vi "PH_ToImage.vi"(0 "Data In":u32[](array[numeric]), 1 "Reset":bool, 2 "Image Array In":i32[][](array[numeric]), 5 "Data Count":i32, 9 "Pixel Time (Laser Pulses)":i32=25, 11 "Trace Bins":i32=25) -> (3 "Image Array Out":i32[][](array[numeric]), 4 "Histograms":i32[][](array[numeric]), 6 "Total Photon Count":u64[](array[numeric]), 8 "Trigger Times":u64[](array[numeric]), 13 "Total Oveflow Count":u64, 14 "Num Records Total":i32, 15 "Traces":i32[][](array[numeric]))   [LabVIEW 2010]
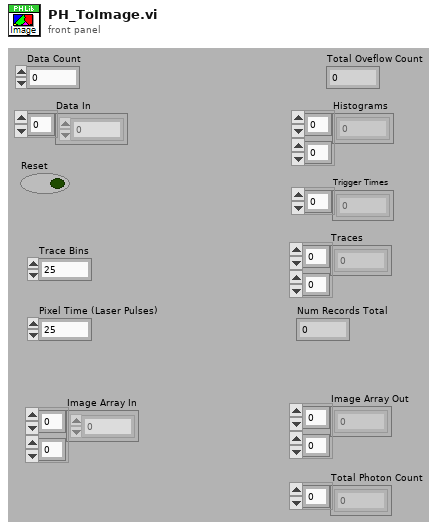
[diagram p1: front panel]
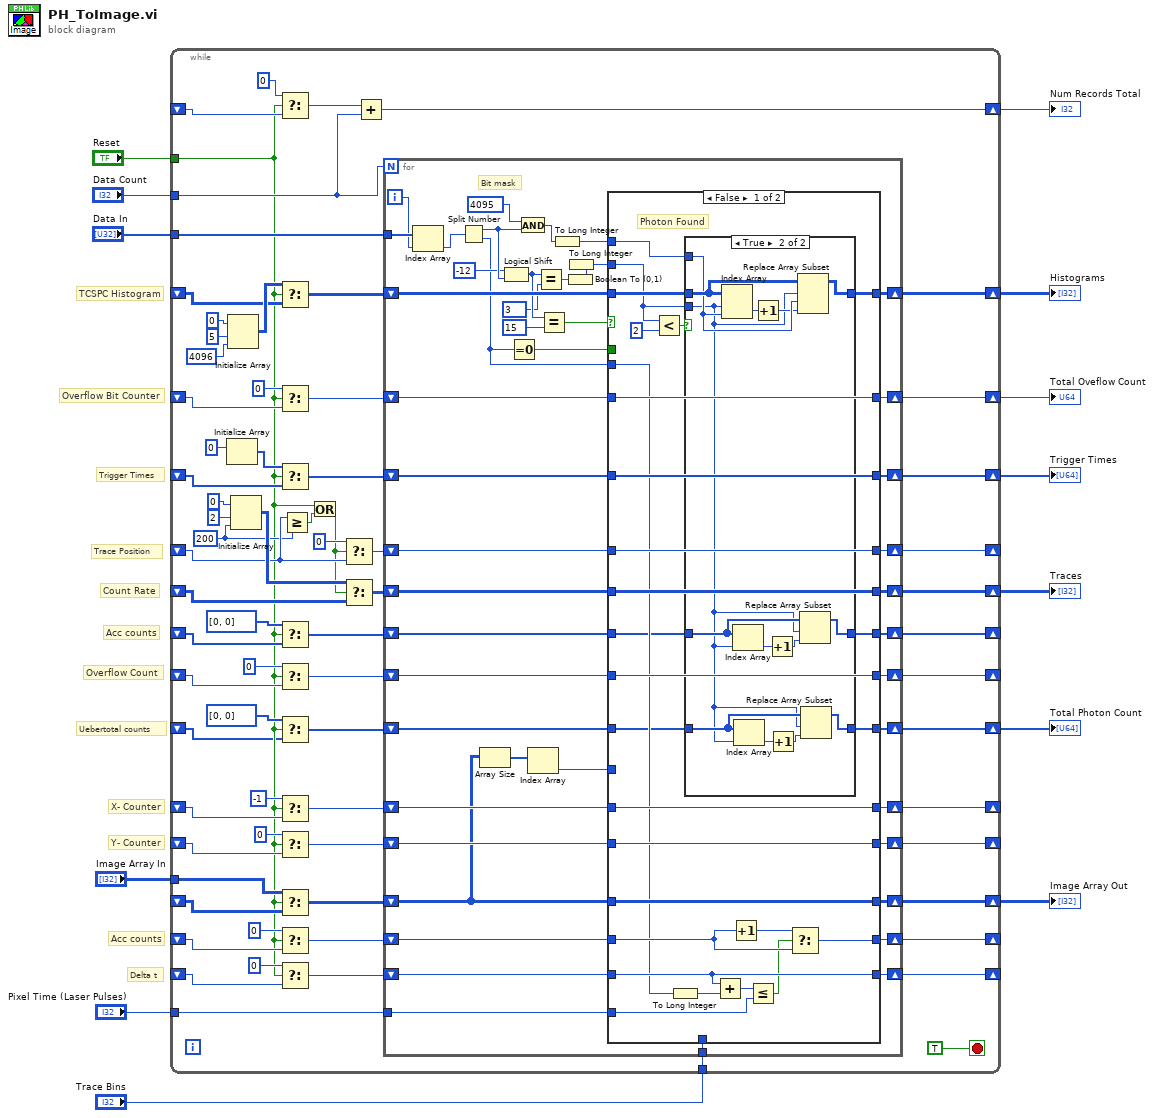
[diagram p0: block diagram]
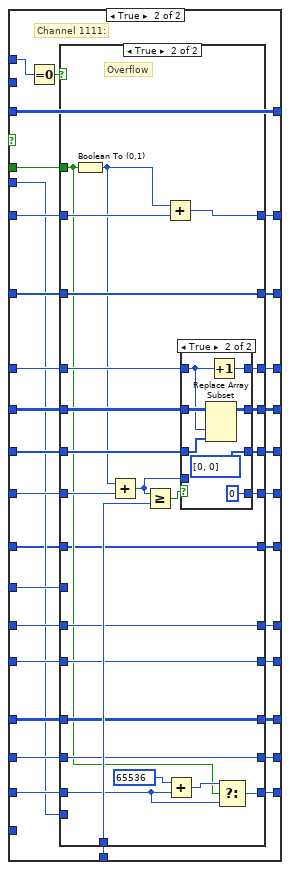
[diagram p3: hidden frame]
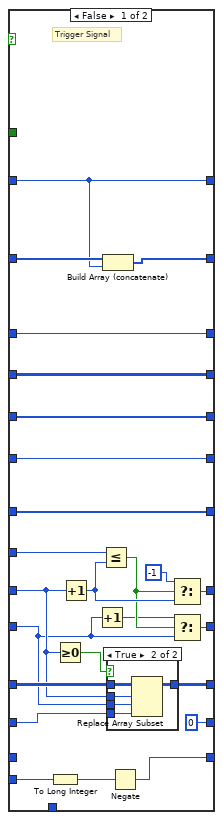
[diagram p4: hidden frame]
diagram:
  # "Uebertotal counts"
  # "Y- Counter"
  # "X- Counter"
  # "Delta t"
  # "Acc counts"
  # "Trace Position"
  # "Overflow Count"
  # "Acc counts"
  # "Count Rate"
  # "Trigger Times"
  # "TCSPC Histogram"
  # "Overflow Bit Counter"
  n1 = while {
    tunnel: "Data In" -> [w82]
    shift-right: [w83] -> w13
    shift-left: _ -> [w78]
    tunnel: "Reset" -> [w17]
    shift-right: [w75] -> w2
    shift-left: _ -> [w74]
    shift-right: [w70] -> w10
    shift-left: _ -> [w69]
    shift-right: [w65] -> w8
    shift-left: _ -> [w64]
    shift-right: [w62] -> _
    shift-left: _ -> [w61]
    shift-right: [w59] -> _
    shift-left: _ -> [w58]
    tunnel: "Trace Bins" -> [w57]
    shift-right: [w54] -> _
    shift-left: _ -> [w52]
    shift-right: [w48] -> w5
    shift-left: _ -> [w47]
    tunnel: "Image Array In" -> [w50]
    shift-right: [w43] -> _
    shift-left: _ -> [w41]
    shift-right: [w42] -> _
    shift-left: _ -> [w40]
    tunnel: "Pixel Time (Laser Pulses)" -> [w39]
    shift-right: [w34] -> _
    shift-left: _ -> [w32]
    shift-right: [w33] -> _
    shift-left: _ -> [w31]
    tunnel: "Data Count" -> [w26]
    shift-right: [w25] -> w3
    shift-left: _ -> [w28]
    shift-right: [w15] -> w1
    shift-left: _ -> [w14]
    stop <- TRUE stop-if-true
    w22 = 200 ("dimension size")
    n2 = Initialize Array(u64 0 ("element")) -> (w72:u64[])  [unwired: 1 in]
    n3 = Initialize Array(0 ("element"), 5 ("dimension size"), 4096 ("dimension size")) -> (w79:i32[][])
    n4 = Initialize Array(0 ("element"), 2 ("dimension size"), w22) -> (w67:i32[][])
    n5 = Select(t=0 ("Data Count 2"), s=w17, f=w28) -> (s? t:f=w27:i32)
    n6 = Select(t=w79, s=w17, f=w78) -> (s? t:f=w80:i32[][])
    n7 = Select(t=u64 0, s=w17, f=w74) -> (s? t:f=w76:u64)
    n8 = Select(t=w72, s=w17, f=w69) -> (s? t:f=w71:u64[])
    n9 = Select(t=u32[] [0, 0] ("initialized array"), s=w17, f=w61) -> (s? t:f=w63:u32[])
    n10 = Select(t=u32 0, s=w17, f=w58) -> (s? t:f=w60:u32)
    n11 = Select(t=u64[] [0, 0] ("initialized array"), s=w17, f=w14) -> (s? t:f=w16:u64[])
    n12 = Select(t=-1, s=w17, f=w32) -> (s? t:f=w36:i32)
    n13 = Select(t=0, s=w17, f=w31) -> (s? t:f=w35:i32)
    n14 = Select(t=w50, s=w17, f=w47) -> (s? t:f=w49:i32[][])
    n15 = Select(t=0, s=w17, f=w41) -> (s? t:f=w45:i32)
    n16 = Select(t=0, s=w17, f=w40) -> (s? t:f=w44:i32)
    n17 = Greater Or Equal?(x=w52, y=w22) -> (x >= y?=w53:bool)
    n18 = Or(x=w17, y=w53) -> (x .or. y?=w51:bool)
    n19 = Select(t=0, s=w51, f=w52) -> (s? t:f=w55:i32)
    n20 = Select(t=w67, s=w51, f=w64) -> (s? t:f=w66:i32[][])
    n21 = Add(x=w27, y=w26) -> (x+y=w25:i32)
    n22 = for {
      N: w26 -> [_]
      tunnel: w82 -> [w94]
      shift-right: [w127] -> w83
      shift-left: w80 -> [w129]
      shift-right: [w121] -> w75
      shift-left: w76 -> [w122]
      shift-right: [w119] -> w70
      shift-left: w71 -> [w120]
      shift-right: [w114] -> w65
      shift-left: w66 -> [w115]
      shift-right: [w116] -> w62
      shift-left: w63 -> [w117]
      shift-right: [w112] -> w59
      shift-left: w60 -> [w113]
      tunnel: w57 -> [w111]
      shift-right: [w109] -> w54
      shift-left: w55 -> [w110]
      shift-right: [w108] -> w48
      shift-left: w49 -> [w100]
      shift-right: [w106] -> w43
      shift-left: w45 -> [w107]
      shift-right: [w104] -> w42
      shift-left: w44 -> [w105]
      tunnel: w39 -> [w96]
      shift-right: [w101] -> w34
      shift-left: w36 -> [w102]
      shift-right: [w97] -> w33
      shift-left: w35 -> [w103]
      shift-right: [w85] -> w15
      shift-left: w16 -> [w86]
      i -> [w93]
      # "Bit mask"
      n23 = Index Array(array=w94, index=w93) -> (element=w92:u32)
      n24 = Split Number(x=w92) -> (hi(x)=w126:u16, lo(x)=w95:u16)
      n25 = Array Size(array=w100) -> (size(s)=w99:i32[])
      n26 = Logical Shift(y=i8 -12, x=w126) -> (x << y=w91:u16)
      n27 = Equal To 0?(x=w95) -> (x = 0?=w118:bool)
      n28 = And(x=u16 4095, y=w126) -> (x .and. y?=w130:u16)
      n29 = Index Array(array=w99) -> (element=w98:i32)  [unwired: 1 in]
      n30 = Equal?(x=w91, y=u16 3) -> (x = y?=w89:bool)
      n31 = Equal?(x=w91, y=u16 15) -> (x = y?=w123:bool)
      n32 = To Long Integer(number=w130) -> (32bit integer=w128:i32)
      n33 = Boolean To (0,1)(Boolean=w89) -> (0, 1=w88:i16)
      n34 = To Long Integer(number=w88) -> (32bit integer=w87:i32)
      n35 = case shown="False" w123 {
        tunnel: w129 -> [w158 w203]
        tunnel: w128 -> [w139 w184]
        tunnel: [w157 w203] -> w127
        tunnel: w87 -> [w135 _]
        tunnel: w122 -> [w156 w205]
        tunnel: [w156 w204] -> w121
        tunnel: w120 -> [w155 w202]
        tunnel: [w155 w201] -> w119
        tunnel: w118 -> [_ w200]
        tunnel: w117 -> [w138 w198]
        tunnel: [w137 w194] -> w116
        tunnel: w115 -> [w154 w197]
        tunnel: [w154 w193] -> w114
        tunnel: w113 -> [w153 w199]
        tunnel: [w153 w195] -> w112
        tunnel: w111 -> [_ w196]
        tunnel: w110 -> [w152 w192]
        tunnel: [w152 w191] -> w109
        tunnel: w100 -> [w151 w189]
        tunnel: [w151 w190] -> w108
        tunnel: w107 -> [w150 w185]
        tunnel: [w149 w186] -> w106
        tunnel: w105 -> [w148 w188]
        tunnel: [w148 w187] -> w104
        tunnel: w103 -> [w147 w183]
        tunnel: w102 -> [w146 w182]
        tunnel: [w146 w181] -> w101
        tunnel: w98 -> [_ w180]
        tunnel: [w147 w179] -> w97
        tunnel: w96 -> [w145 _]
        tunnel: w95 -> [w141 w178]
        tunnel: w86 -> [w133 w177]
        tunnel: [w132 w176] -> w85
        frame False {
          # "Photon Found"
          n36 = Less?(x=w135, y=2) -> (x < y?=w136:bool)
          n37 = To Long Integer(number=w141) -> (32bit integer=w140:i32)
          n38 = case shown="True" w136 {
            tunnel: w158 -> [w161 w175]
            tunnel: [w161 w174] -> w157
            tunnel: w139 -> [_ w173]
            tunnel: w135 -> [_ w162]
            tunnel: w138 -> [w160 w172]
            tunnel: [w160 w171] -> w137
            tunnel: w133 -> [w159 w164]
            tunnel: [w159 w163] -> w132
            frame False {
            }
            frame True {
              n39 = Index Array(array=w175, index (row)=w162, index (col)=w173) -> (element=w170:i32)
              n40 = Index Array(array=w172, index=w162) -> (element=w168:u32)
              n41 = Index Array(array=w164, index=w162) -> (element=w166:u64)
              n42 = Increment(x=w170) -> (x+1=w169:i32)
              n43 = Increment(x=w168) -> (x+1=w167:u32)
              n44 = Increment(x=w166) -> (x+1=w165:u64)
              n45 = Replace Array Subset(array=w175, new element=w169, index (row)=w162, index (col)=w173) -> (w174:i32[][])
              n46 = Replace Array Subset(array=w172, new element=w167, index=w162) -> (w171:u32[])
              n47 = Replace Array Subset(array=w164, new element=w165, index=w162) -> (w163:u64[])
            }
          }
          n48 = Add(x=w148, y=w140) -> (x+y=w142:i32)
          n49 = Increment(x=w150) -> (x+1=w144:i32)
          n50 = Less Or Equal?(x=w142, y=w145) -> (x <= y?=w143:bool)
          n51 = Select(t=w144, s=w143, f=w150) -> (s? t:f=w149:i32)
        }
        frame True {
          # "Channel 1111:"
          n52 = Equal To 0?(x=w184) -> (x = 0?=w206:bool)
          n53 = case shown="True" w206 {
            tunnel: w205 -> [w229 w261]
            tunnel: [w229 w260] -> w204
            tunnel: w202 -> [w231 w262]
            tunnel: [w230 w262] -> w201
            tunnel: w200 -> [_ w239]
            tunnel: w199 -> [w228 w245]
            tunnel: w198 -> [w227 w256]
            tunnel: w197 -> [w226 w254]
            tunnel: w196 -> [_ w259]
            tunnel: [w228 w257] -> w195
            tunnel: [w227 w255] -> w194
            tunnel: [w226 w253] -> w193
            tunnel: w192 -> [w225 w252]
            tunnel: [w225 w251] -> w191
            tunnel: [w222 w250] -> w190
            tunnel: w189 -> [w223 w250]
            tunnel: w188 -> [_ w240]
            tunnel: [w208 w241] -> w187
            tunnel: [0 ("t") w248] -> w186
            tunnel: w185 -> [w221 w248]
            tunnel: w178 -> [w224 _]
            tunnel: w183 -> [w211 w247]
            tunnel: w182 -> [w216 w246]
            tunnel: [w218 w246] -> w181
            tunnel: w180 -> [w217 _]
            tunnel: [w212 w247] -> w179
            tunnel: w177 -> [w207 w238]
            tunnel: [w207 w238] -> w176
            frame False {
              # "Trigger Signal"
              n54 = To Long Integer(number=w224) -> (32bit integer=w209:i32)
              n55 = Greater Or Equal To 0?(x=w216) -> (x >= 0?=w219:bool)
              n56 = Increment(x=w216) -> (x+1=w215:i32)
              n57 = Increment(x=w211) -> (x+1=w210:i32)
              n58 = Less Or Equal?(x=w217, y=w215) -> (x <= y?=w213:bool)
              n59 = Build Array (concatenate)(w231, w229) -> (w230:u64[])
              n60 = case shown="True" w219 {
                tunnel: w223 -> [w232 w237]
                tunnel: [w232 w236] -> w222
                tunnel: w221 -> [_ w235]
                tunnel: w211 -> [_ w234]
                tunnel: w216 -> [_ w233]
                frame False {
                }
                frame True {
                  n61 = Replace Array Subset(array=w237, new element=w235, index (row)=w233, index (col)=w234) -> (w236:i32[][])
                }
              }
              n62 = Negate(x=w209) -> (-x=w208:i32)
              n63 = Select(t=-1, s=w213, f=w215) -> (s? t:f=w218:i32)
              n64 = Select(t=w210, s=w213, f=w211) -> (s? t:f=w212:i32)
            }
            frame True {
              # "Overflow"
              n65 = Boolean To (0,1)(Boolean=w239) -> (0, 1=w243:i16)
              n66 = Add(x=w243, y=w245) -> (x+y=w244:u32)
              n67 = Greater Or Equal?(x=w244, y=w259) -> (x >= y?=w258:bool)
              n68 = Add(x=w243, y=w261) -> (x+y=w260:u64)
              n69 = Add(x=65536 ("t"), y=w240) -> (x+y=w242:i32)
              n70 = case shown="True" w258 {
                tunnel: w244 -> [w266 _]
                tunnel: [w266 u32 0] -> w257
                tunnel: w256 -> [w265 w271]
                tunnel: [w265 u32[] [0, 0] ("initialized array")] -> w255
                tunnel: w254 -> [w264 w272]
                tunnel: [w264 w270] -> w253
                tunnel: w252 -> [w263 w268]
                tunnel: [w263 w269] -> w251
                frame False {
                }
                frame True {
                  n71 = Replace Array Subset(array=w272, new element=w271, index (col)=w268) -> (w270:i32[][])  [unwired: 1 in]
                  n72 = Increment(x=w268) -> (x+1=w269:i32)
                }
              }
              n73 = Select(t=w242, s=w239, f=w240) -> (s? t:f=w241:i32)
            }
          }
        }
      }
    }
  }
  "Histograms" <- w13
  "Trigger Times" <- w10
  "Traces" <- w8
  "Image Array Out" <- w5
  "Num Records Total" <- w3
  "Total Oveflow Count" <- w2
  "Total Photon Count" <- w1
